vi "Fetch Measurement - Single point.vi"(8 "error in":errorcluster, 11 "Single point perform measurement":T1={"Source Ganged Session Out"={"Ganged Config"=enum."Series", "Session List"=[], "Session Mode"=[], "Channel"=[]}, "Load Ganged Session Out"={"Ganged Config"=enum."Series", "Session List"=[], "Session Mode"=[], "Channel"=[]}, "Source Measure Record Length"=0, "Load Measure Record Length"=0, "Measurement Results"={"dt"=[], "Source voltages"=[], "Source currents"=[], "Load voltages"=[], "Load currents"=[], "Ganged source voltages"=[], "Ganged source currents"=[], "Ganged load voltages"=[], "Ganged load currents"=[], "Mean values"=[], "Minimum values"=[], "Maximum values"=[], "Status"="", "Eload status"=""}, "Load Slave resource name"=[], "Load Master/Single resource name"="", "Source Slave resource name"=[], "Source Master/Single resource name"="", "Load ganged/single"=FALSE, "Source ganged/single"=FALSE, "Source channel name"="", "Load channel name"="", "Source session out"="", "Load session out"="", "Number of Eload used"=0, "Load Source ON/OFF"=enum."SOURCE ON", "Measurement timeout"=0.0}) -> (0 "error out":errorcluster, 3 "Single point perform measurement":T1={"Source Ganged Session Out"={"Ganged Config"=enum."Series", "Session List"=[], "Session Mode"=[], "Channel"=[]}, "Load Ganged Session Out"={"Ganged Config"=enum."Series", "Session List"=[], "Session Mode"=[], "Channel"=[]}, "Source Measure Record Length"=0, "Load Measure Record Length"=0, "Measurement Results"={"dt"=[], "Source voltages"=[], "Source currents"=[], "Load voltages"=[], "Load currents"=[], "Ganged source voltages"=[], "Ganged source currents"=[], "Ganged load voltages"=[], "Ganged load currents"=[], "Mean values"=[], "Minimum values"=[], "Maximum values"=[], "Status"="", "Eload status"=""}, "Load Slave resource name"=[], "Load Master/Single resource name"="", "Source Slave resource name"=[], "Source Master/Single resource name"="", "Load ganged/single"=FALSE, "Source ganged/single"=FALSE, "Source channel name"="", "Load channel name"="", "Source session out"="", "Load session out"="", "Number of Eload used"=0, "Load Source ON/OFF"=enum."SOURCE ON", "Measurement timeout"=0.0})   [LabVIEW 2021, in "Single Point_Channel Ganging.lvlib"]
doc: "This VI will fetch the measurement for different configuration for Single Point measurement"
uses:
  Single Point_Channel Ganging.lvlib
  Controls/Perform measurement-control.ctl
  shared subVIs/ctl/NIDCPower_channel_ganging - ctl - ganged session.ctl
  shared subVIs/ctl/NIDCPower_channel_ganging - ctl - ganged config.ctl
  shared subVIs/ctl/NIDCPower_channel_ganging - ctl - channel mode.ctl
  Measurement Results.ctl
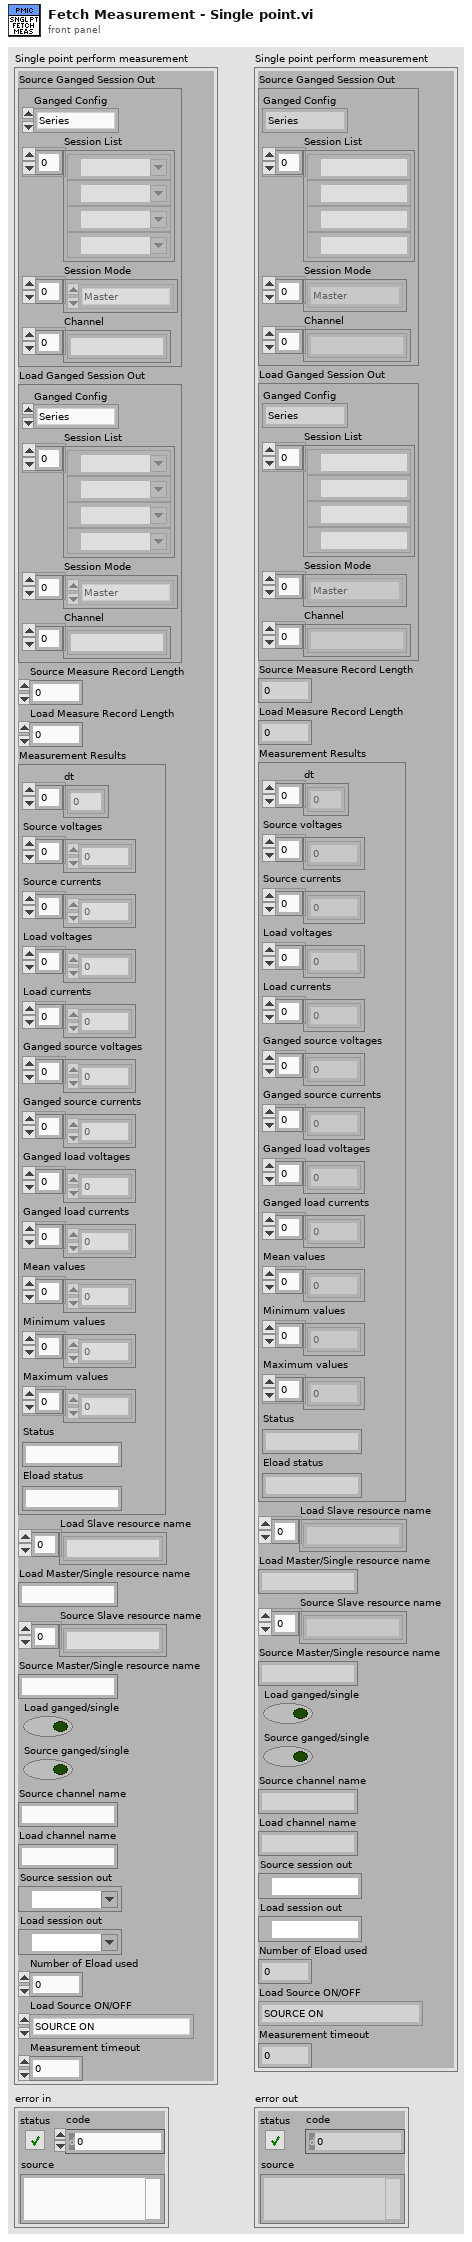
[diagram p1: front panel]
types:
  T1 = typedef "Single Point_Channel Ganging.lvlib/Perform measurement-control.ctl" = cluster{"Source Ganged Session Out":T2, "Load Ganged Session Out":T2, "Source Measure Record Length":i32, "Load Measure Record Length":i32, "Measurement Results":T5, "Load Slave resource name":string[], "Load Master/Single resource name":string, "Source Slave resource name":string[], "Source Master/Single resource name":string, "Load ganged/single":bool, "Source ganged/single":bool, "Source channel name":string, "Load channel name":string, "Source session out":refnum<k15>, "Load session out":refnum<k15>, "Number of Eload used":i32, "Load Source ON/OFF":enum16{"SOURCE AND LOAD OFF", "SOURCE ON", "LOAD ON", "SOURCE AND LOAD ON"}, "Measurement timeout":dbl}
  T2 = typedef "NIDCPower_channel_ganging - ctl - ganged session.ctl" = cluster{"Ganged Config":T3, "Session List":refnum<k15>[], "Session Mode":T4[], "Channel":string[]}
  T3 = typedef "NIDCPower_channel_ganging - ctl - ganged config.ctl" = enum32{"Series", "Parallel", "Manual"}
  T4 = typedef "NIDCPower_channel_ganging - ctl - channel mode.ctl" = enum32{"Master", "Slave", "Slave - Inverted"}
  T5 = typedef "Single Point_Channel Ganging.lvlib/Measurement Results.ctl" = cluster{"dt":dbl[], "Source voltages":dbl[], "Source currents":dbl[], "Load voltages":dbl[], "Load currents":dbl[], "Ganged source voltages":dbl[], "Ganged source currents":dbl[], "Ganged load voltages":dbl[], "Ganged load currents":dbl[], "Mean values":dbl[], "Minimum values":dbl[], "Maximum values":dbl[], "Status":string, "Eload status":string}
  T6 = enum16{"SOURCE AND LOAD OFF", "SOURCE ON", "LOAD ON", "SOURCE AND LOAD ON"}
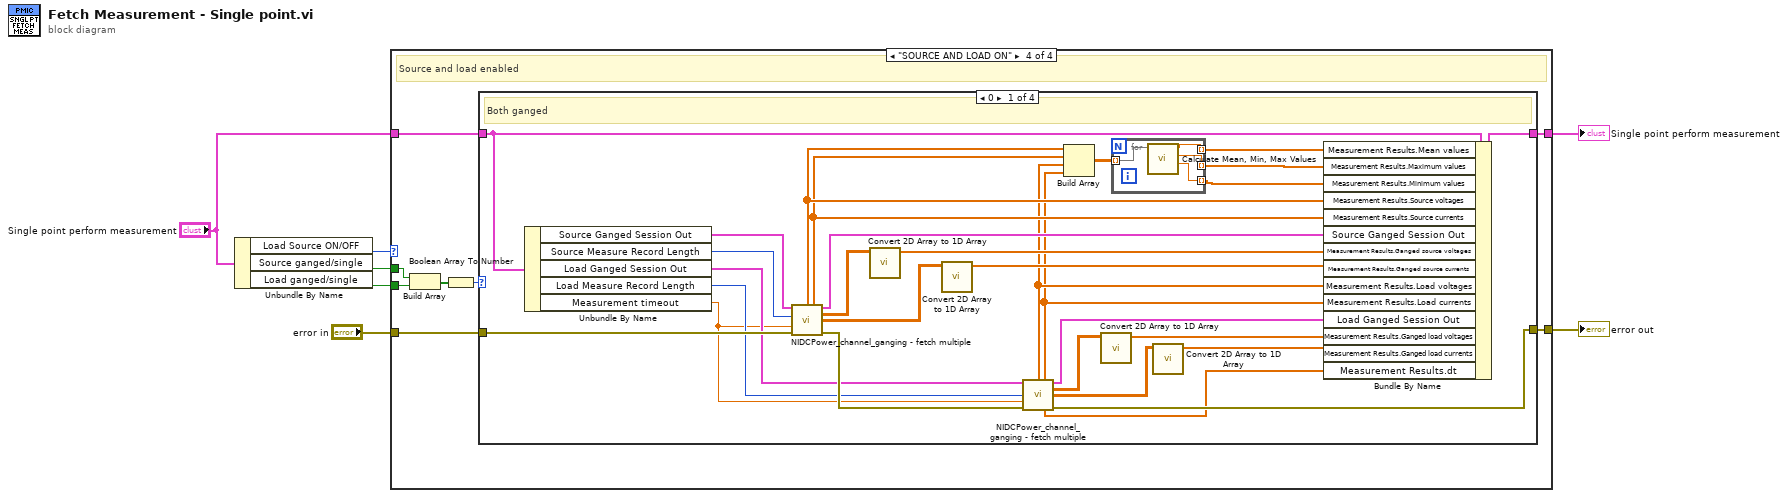
[diagram p0: block diagram]
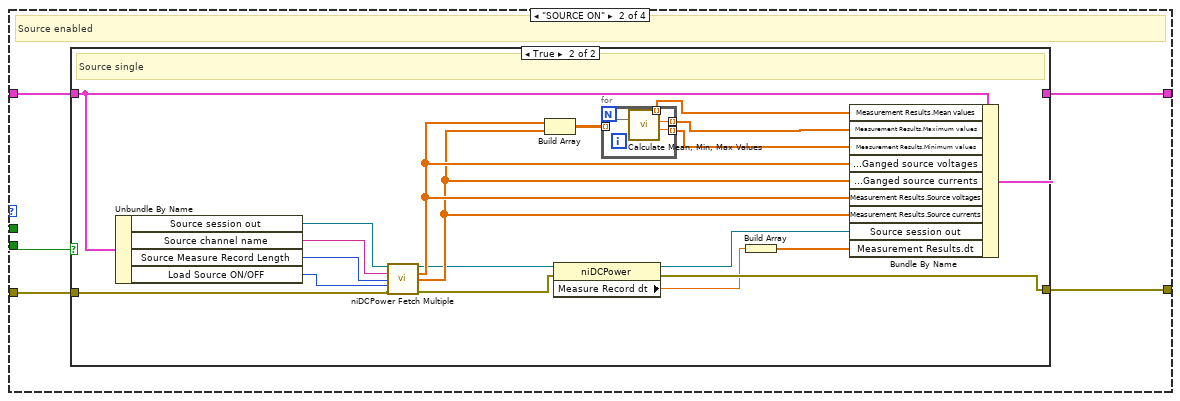
[diagram p3: hidden frame]
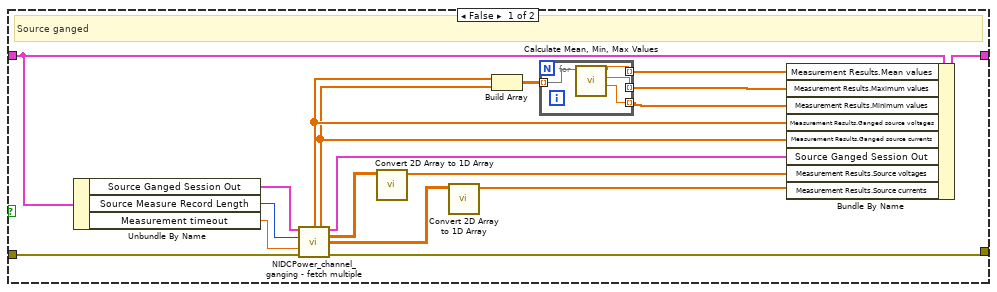
[diagram p4: hidden frame]
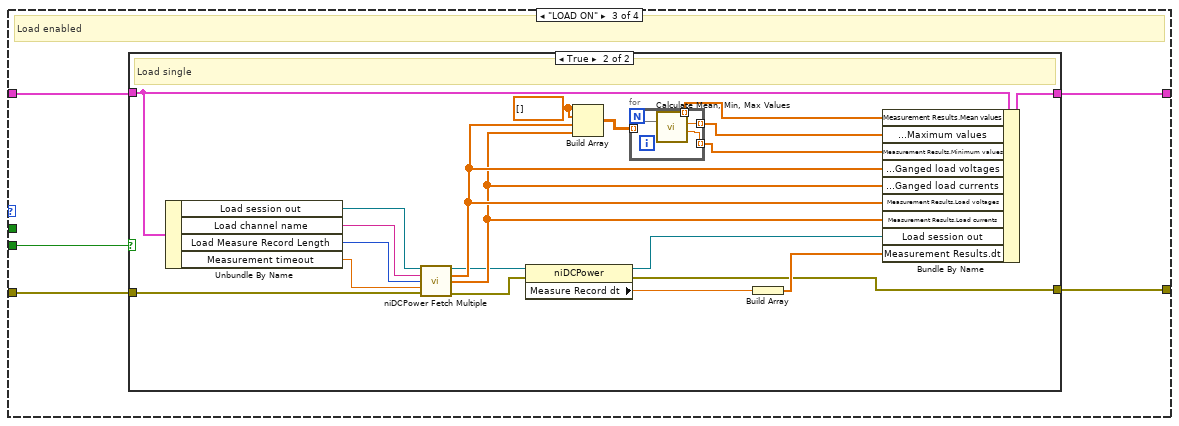
[diagram p5: hidden frame]
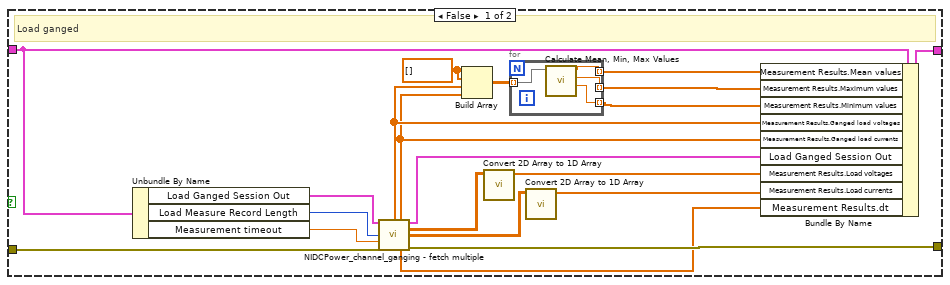
[diagram p6: hidden frame]
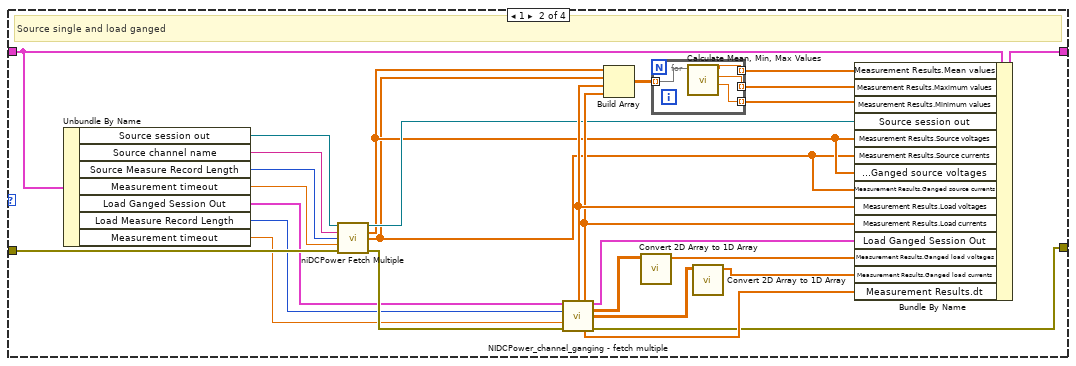
[diagram p7: hidden frame]
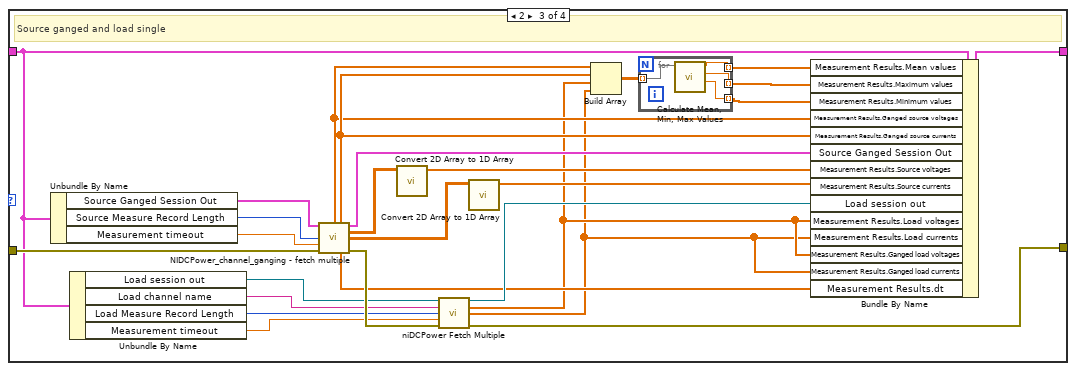
[diagram p8: hidden frame]
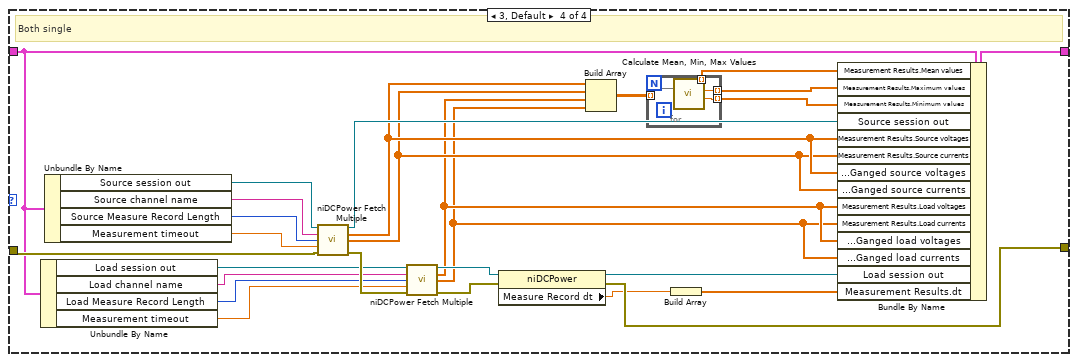
[diagram p9: hidden frame]
diagram:
  n1 = Unbundle By Name("Single point perform measurement") -> ("Load Source ON/OFF"=w5:T6, "Source ganged/single"=w6:bool, "Load ganged/single"=w7:bool)
  n2 = case shown="\"SOURCE AND LOAD ON\"" w5 {
    tunnel: "error in" -> [w8 w14 w64 w120]
    tunnel: [w9 w10 w60 w119] -> w2
    tunnel: [w8 w11 w61 w118] -> w3
    tunnel: "Single point perform measurement" -> [w9 w12 w63 w117]
    tunnel: w6 -> [_ w13 _ w115]
    tunnel: w7 -> [_ _ w62 w114]
    frame Default {
    }
    frame "SOURCE ON" {
      # "Source enabled"
      n3 = case shown="True" w13 {
        tunnel: w12 -> [w32 w55]
        tunnel: w14 -> [w30 w49]
        tunnel: [w29 w54] -> w10
        tunnel: [w16 w46] -> w11
        frame False {
          # "Source ganged"
          n4 = Unbundle By Name(w32) -> ("Source Ganged Session Out"=w31:T2, "Source Measure Record Length"=w27:i32, "Measurement timeout"=w15:dbl)
          n5 = call "NIDCPower_channel_ganging - fetch multiple.vi"("Ganged Session In"=w31, "Count"=w27, "timeout (1.0)"=w15, "error in (no error)"=w30) -> ("Ganged Voltage Measurement"=w22:dbl[], "Ganged Current Measurement"=w21:dbl[], "Ganged Session Out"=w28:T2, "voltage measurements"=w26:dbl[][], "current measurements"=w23:dbl[][], "error out"=w16:errorcluster)  [unwired: 4 in, 2 out]
          n6 = call "Convert 2D Array to 1D Array.vi"("Array in"=w26) -> ("Array out"=w25:dbl[])  [unwired: 10 in]
          n7 = call "Convert 2D Array to 1D Array.vi"("Array in"=w23) -> ("Array out"=w24:dbl[])  [unwired: 10 in]
          n8 = Build Array(w22, w21) -> (w20:dbl[][])
          n9 = for {
            tunnel: w20 -> [w36] mode=indexing
            tunnel: [w35] -> w19 mode=indexing
            tunnel: [w34] -> w18 mode=indexing
            tunnel: [w33] -> w17 mode=indexing
            n10 = call "Calculate Mean, Min, Max Values.vi"("Ganged Measurement"=w36) -> ("Min value"=w33:dbl, "Max value"=w34:dbl, "Mean value"=w35:dbl)  [unwired: 8 in]
          }
          n11 = Bundle By Name(cluster=w32, "Measurement Results.Mean values"=w19, "Measurement Results.Maximum values"=w18, "Measurement Results.Minimum values"=w17, "Measurement Results.Ganged source voltages"=w22, "Measurement Results.Ganged source currents"=w21, "Source Ganged Session Out"=w28, "Measurement Results.Source voltages"=w25, "Measurement Results.Source currents"=w24) -> (w29:T1)
        }
        frame True {
          # "Source single"
          n12 = Unbundle By Name(w55) -> ("Source session out"=w48:refnum<k15>, "Source channel name"=w39:string, "Source Measure Record Length"=w40:i32, "Load Source ON/OFF"=w37:T6)
          n13 = call <instrlib>:"niDCPower Fetch Multiple.vi"("instrument handle"=w48, "channel name"=w39, "count (1)"=w40, "timeout (1.0)"=w37, "error in (no error)"=w49) -> ("instrument handle out"=w42:refnum<k15>, "voltage measurements"=w47:dbl[], "current measurements"=w44:dbl[], "error out"=w43:errorcluster)  [unwired: 7 out]
          n14 = Build Array(w47, w44) -> (w53:dbl[][])
          n15 = property class="niDCPower"(reference=w42, error in=w43) -> (reference out=w38:refnum<k15>, error out=w46:errorcluster, "Measure Record dt"=w45:dbl)
          n16 = for {
            tunnel: w53 -> [w59] mode=indexing
            tunnel: [w58] -> w52 mode=indexing
            tunnel: [w57] -> w51 mode=indexing
            tunnel: [w56] -> w50 mode=indexing
            n17 = call "Calculate Mean, Min, Max Values.vi"("Ganged Measurement"=w59) -> ("Min value"=w56:dbl, "Max value"=w57:dbl, "Mean value"=w58:dbl)  [unwired: 8 in]
          }
          n18 = Build Array(w45) -> (w41:dbl[])
          n19 = Bundle By Name(cluster=w55, "Measurement Results.Mean values"=w52, "Measurement Results.Maximum values"=w51, "Measurement Results.Minimum values"=w50, "Measurement Results.Ganged source voltages"=w47, "Measurement Results.Ganged source currents"=w44, "Measurement Results.Source voltages"=w47, "Measurement Results.Source currents"=w44, "Source session out"=w38, "Measurement Results.dt"=w41) -> (w54:T1)
        }
      }
    }
    frame "LOAD ON" {
      # "Load enabled"
      n20 = case shown="True" w62 {
        tunnel: w63 -> [w84 w104]
        tunnel: w64 -> [w68 w93]
        tunnel: [w82 w103] -> w60
        tunnel: [w81 w90] -> w61
        frame False {
          w65 = dbl[] [] ("element")
          # "Load ganged"
          n21 = Unbundle By Name(w84) -> ("Load Ganged Session Out"=w83:T2, "Load Measure Record Length"=w66:i32, "Measurement timeout"=w67:dbl)
          n22 = call "NIDCPower_channel_ganging - fetch multiple.vi"("Ganged Session In"=w83, "Count"=w66, "timeout (1.0)"=w67, "error in (no error)"=w68) -> ("Ganged Voltage Measurement"=w74:dbl[], "Ganged Current Measurement"=w73:dbl[], "Ganged Session Out"=w80:T2, "voltage measurements"=w78:dbl[][], "current measurements"=w76:dbl[][], "Measure Record dt"=w79:dbl[], "error out"=w81:errorcluster)  [unwired: 4 in, 1 out]
          n23 = Build Array(w65, w65, w74, w73) -> (w72:dbl[][])
          n24 = call "Convert 2D Array to 1D Array.vi"("Array in"=w78) -> ("Array out"=w77:dbl[])  [unwired: 10 in]
          n25 = for {
            tunnel: w72 -> [w88] mode=indexing
            tunnel: [w87] -> w71 mode=indexing
            tunnel: [w86] -> w70 mode=indexing
            tunnel: [w85] -> w69 mode=indexing
            n26 = call "Calculate Mean, Min, Max Values.vi"("Ganged Measurement"=w88) -> ("Min value"=w85:dbl, "Max value"=w86:dbl, "Mean value"=w87:dbl)  [unwired: 8 in]
          }
          n27 = call "Convert 2D Array to 1D Array.vi"("Array in"=w76) -> ("Array out"=w75:dbl[])  [unwired: 10 in]
          n28 = Bundle By Name(cluster=w84, "Measurement Results.Mean values"=w71, "Measurement Results.Maximum values"=w70, "Measurement Results.Minimum values"=w69, "Measurement Results.Ganged load voltages"=w74, "Measurement Results.Ganged load currents"=w73, "Load Ganged Session Out"=w80, "Measurement Results.Load voltages"=w77, "Measurement Results.Load currents"=w75, "Measurement Results.dt"=w79) -> (w82:T1)
        }
        frame True {
          w89 = dbl[] [] ("element")
          # "Load single"
          n29 = Unbundle By Name(w104) -> ("Load session out"=w108:refnum<k15>, "Load channel name"=w107:string, "Load Measure Record Length"=w94:i32, "Measurement timeout"=w91:dbl)
          n30 = call <instrlib>:"niDCPower Fetch Multiple.vi"("instrument handle"=w108, "channel name"=w107, "count (1)"=w94, "timeout (1.0)"=w91, "error in (no error)"=w93) -> ("instrument handle out"=w97:refnum<k15>, "voltage measurements"=w106:dbl[], "current measurements"=w105:dbl[], "error out"=w98:errorcluster)  [unwired: 7 out]
          n31 = property class="niDCPower"(reference=w97, error in=w98) -> (reference out=w92:refnum<k15>, error out=w90:errorcluster, "Measure Record dt"=w96:dbl)
          n32 = Build Array(w89, w89, w106, w105) -> (w102:dbl[][])
          n33 = for {
            tunnel: w102 -> [w112] mode=indexing
            tunnel: [w111] -> w101 mode=indexing
            tunnel: [w110] -> w100 mode=indexing
            tunnel: [w109] -> w99 mode=indexing
            n34 = call "Calculate Mean, Min, Max Values.vi"("Ganged Measurement"=w112) -> ("Min value"=w109:dbl, "Max value"=w110:dbl, "Mean value"=w111:dbl)  [unwired: 8 in]
          }
          n35 = Build Array(w96) -> (w95:dbl[])
          n36 = Bundle By Name(cluster=w104, "Measurement Results.Mean values"=w101, "Measurement Results.Maximum values"=w100, "Measurement Results.Minimum values"=w99, "Measurement Results.Ganged load voltages"=w106, "Measurement Results.Ganged load currents"=w105, "Measurement Results.Load voltages"=w106, "Measurement Results.Load currents"=w105, "Load session out"=w92, "Measurement Results.dt"=w95) -> (w103:T1)
        }
      }
    }
    frame "SOURCE AND LOAD ON" {
      # "Source and load enabled"
      n37 = Build Array(w115, w114) -> (w116:bool[])
      n38 = Boolean Array To Number(Boolean array=w116) -> (number=w113:u32)
      n39 = case shown="0" w113 {
        tunnel: w117 -> [w149 w160 w192 w228]
        tunnel: w120 -> [w146 w167 w199 w236]
        tunnel: [w144 w168 w198 w242] -> w119
        tunnel: [w143 w156 w196 w231] -> w118
        frame 0 {
          # "Both ganged"
          n40 = Unbundle By Name(w149) -> ("Source Ganged Session Out"=w148:T2, "Source Measure Record Length"=w123:i32, "Load Ganged Session Out"=w145:T2, "Load Measure Record Length"=w122:i32, "Measurement timeout"=w121:dbl)
          n41 = call "NIDCPower_channel_ganging - fetch multiple.vi"("Ganged Session In"=w148, "Count"=w123, "timeout (1.0)"=w121, "error in (no error)"=w146) -> ("Ganged Voltage Measurement"=w131:dbl[], "Ganged Current Measurement"=w130:dbl[], "Ganged Session Out"=w142:T2, "voltage measurements"=w139:dbl[][], "current measurements"=w136:dbl[][], "error out"=w147:errorcluster)  [unwired: 4 in, 2 out]
          n42 = call "Convert 2D Array to 1D Array.vi"("Array in"=w139) -> ("Array out"=w138:dbl[])  [unwired: 10 in]
          n43 = call "Convert 2D Array to 1D Array.vi"("Array in"=w136) -> ("Array out"=w137:dbl[])  [unwired: 10 in]
          n44 = call "NIDCPower_channel_ganging - fetch multiple.vi"("Ganged Session In"=w145, "Count"=w122, "timeout (1.0)"=w121, "error in (no error)"=w147) -> ("Ganged Voltage Measurement"=w129:dbl[], "Ganged Current Measurement"=w128:dbl[], "Ganged Session Out"=w141:T2, "voltage measurements"=w135:dbl[][], "current measurements"=w133:dbl[][], "Measure Record dt"=w140:dbl[], "error out"=w143:errorcluster)  [unwired: 4 in, 1 out]
          n45 = Build Array(w131, w130, w129, w128) -> (w127:dbl[][])
          n46 = call "Convert 2D Array to 1D Array.vi"("Array in"=w135) -> ("Array out"=w134:dbl[])  [unwired: 10 in]
          n47 = for {
            tunnel: w127 -> [w153] mode=indexing
            tunnel: [w152] -> w126 mode=indexing
            tunnel: [w151] -> w125 mode=indexing
            tunnel: [w150] -> w124 mode=indexing
            n48 = call "Calculate Mean, Min, Max Values.vi"("Ganged Measurement"=w153) -> ("Min value"=w150:dbl, "Max value"=w151:dbl, "Mean value"=w152:dbl)  [unwired: 8 in]
          }
          n49 = call "Convert 2D Array to 1D Array.vi"("Array in"=w133) -> ("Array out"=w132:dbl[])  [unwired: 10 in]
          n50 = Bundle By Name(cluster=w149, "Measurement Results.Mean values"=w126, "Measurement Results.Maximum values"=w125, "Measurement Results.Minimum values"=w124, "Measurement Results.Source voltages"=w131, "Measurement Results.Source currents"=w130, "Source Ganged Session Out"=w142, "Measurement Results.Ganged source voltages"=w138, "Measurement Results.Ganged source currents"=w137, "Measurement Results.Load voltages"=w129, "Measurement Results.Load currents"=w128, "Load Ganged Session Out"=w141, "Measurement Results.Ganged load voltages"=w134, "Measurement Results.Ganged load currents"=w132, "Measurement Results.dt"=w140) -> (w144:T1)
        }
        frame 1 {
          # "Source single and load ganged"
          n51 = Unbundle By Name(w160) -> ("Source session out"=w165:refnum<k15>, "Source channel name"=w162:string, "Source Measure Record Length"=w164:i32, "Measurement timeout"=w159:dbl, "Load Ganged Session Out"=w158:T2, "Load Measure Record Length"=w161:i32, "Measurement timeout"=w157:dbl)
          n52 = call <instrlib>:"niDCPower Fetch Multiple.vi"("instrument handle"=w165, "channel name"=w162, "count (1)"=w164, "timeout (1.0)"=w159, "error in (no error)"=w167) -> ("instrument handle out"=w163:refnum<k15>, "voltage measurements"=w155:dbl[], "current measurements"=w154:dbl[], "error out"=w166:errorcluster)  [unwired: 7 out]
          n53 = call "NIDCPower_channel_ganging - fetch multiple.vi"("Ganged Session In"=w158, "Count"=w161, "timeout (1.0)"=w157, "error in (no error)"=w166) -> ("Ganged Voltage Measurement"=w174:dbl[], "Ganged Current Measurement"=w173:dbl[], "Ganged Session Out"=w180:T2, "voltage measurements"=w178:dbl[][], "current measurements"=w176:dbl[][], "Measure Record dt"=w179:dbl[], "error out"=w156:errorcluster)  [unwired: 4 in, 1 out]
          n54 = Build Array(w155, w154, w174, w173) -> (w172:dbl[][])
          n55 = call "Convert 2D Array to 1D Array.vi"("Array in"=w178) -> ("Array out"=w177:dbl[])  [unwired: 10 in]
          n56 = for {
            tunnel: w172 -> [w184] mode=indexing
            tunnel: [w183] -> w171 mode=indexing
            tunnel: [w182] -> w170 mode=indexing
            tunnel: [w181] -> w169 mode=indexing
            n57 = call "Calculate Mean, Min, Max Values.vi"("Ganged Measurement"=w184) -> ("Min value"=w181:dbl, "Max value"=w182:dbl, "Mean value"=w183:dbl)  [unwired: 8 in]
          }
          n58 = call "Convert 2D Array to 1D Array.vi"("Array in"=w176) -> ("Array out"=w175:dbl[])  [unwired: 10 in]
          n59 = Bundle By Name(cluster=w160, "Measurement Results.Mean values"=w171, "Measurement Results.Maximum values"=w170, "Measurement Results.Minimum values"=w169, "Source session out"=w163, "Measurement Results.Source voltages"=w155, "Measurement Results.Source currents"=w154, "Measurement Results.Ganged source voltages"=w155, "Measurement Results.Ganged source currents"=w154, "Measurement Results.Load voltages"=w174, "Measurement Results.Load currents"=w173, "Load Ganged Session Out"=w180, "Measurement Results.Ganged load voltages"=w177, "Measurement Results.Ganged load currents"=w175, "Measurement Results.dt"=w179) -> (w168:T1)
        }
        frame 2 {
          # "Source ganged and load single"
          n60 = Unbundle By Name(w192) -> ("Source Ganged Session Out"=w200:T2, "Source Measure Record Length"=w194:i32, "Measurement timeout"=w187:dbl)
          n61 = Unbundle By Name(w192) -> ("Load session out"=w191:refnum<k15>, "Load channel name"=w190:string, "Load Measure Record Length"=w189:i32, "Measurement timeout"=w188:dbl)
          n62 = call "NIDCPower_channel_ganging - fetch multiple.vi"("Ganged Session In"=w200, "Count"=w194, "timeout (1.0)"=w187, "error in (no error)"=w199) -> ("Ganged Voltage Measurement"=w206:dbl[], "Ganged Current Measurement"=w207:dbl[], "Ganged Session Out"=w201:T2, "voltage measurements"=w202:dbl[][], "current measurements"=w205:dbl[][], "Measure Record dt"=w193:dbl[], "error out"=w197:errorcluster)  [unwired: 4 in, 1 out]
          n63 = call "Convert 2D Array to 1D Array.vi"("Array in"=w202) -> ("Array out"=w203:dbl[])  [unwired: 10 in]
          n64 = call <instrlib>:"niDCPower Fetch Multiple.vi"("instrument handle"=w191, "channel name"=w190, "count (1)"=w189, "timeout (1.0)"=w188, "error in (no error)"=w197) -> ("instrument handle out"=w195:refnum<k15>, "voltage measurements"=w186:dbl[], "current measurements"=w185:dbl[], "error out"=w196:errorcluster)  [unwired: 7 out]
          n65 = call "Convert 2D Array to 1D Array.vi"("Array in"=w205) -> ("Array out"=w204:dbl[])  [unwired: 10 in]
          n66 = Build Array(w206, w207, w186, w185) -> (w208:dbl[][])
          n67 = for {
            tunnel: w208 -> [w215] mode=indexing
            tunnel: [w214] -> w209 mode=indexing
            tunnel: [w213] -> w210 mode=indexing
            tunnel: [w212] -> w211 mode=indexing
            n68 = call "Calculate Mean, Min, Max Values.vi"("Ganged Measurement"=w215) -> ("Min value"=w212:dbl, "Max value"=w213:dbl, "Mean value"=w214:dbl)  [unwired: 8 in]
          }
          n69 = Bundle By Name(cluster=w192, "Measurement Results.Mean values"=w209, "Measurement Results.Maximum values"=w210, "Measurement Results.Minimum values"=w211, "Measurement Results.Ganged source voltages"=w206, "Measurement Results.Ganged source currents"=w207, "Source Ganged Session Out"=w201, "Measurement Results.Source voltages"=w203, "Measurement Results.Source currents"=w204, "Load session out"=w195, "Measurement Results.Load voltages"=w186, "Measurement Results.Load currents"=w185, "Measurement Results.Ganged load voltages"=w186, "Measurement Results.Ganged load currents"=w185, "Measurement Results.dt"=w193) -> (w198:T1)
        }
        frame 3, Default {
          # "Both single"
          n70 = Unbundle By Name(w228) -> ("Load session out"=w227:refnum<k15>, "Load channel name"=w226:string, "Load Measure Record Length"=w225:i32, "Measurement timeout"=w220:dbl)
          n71 = Unbundle By Name(w228) -> ("Source session out"=w235:refnum<k15>, "Source channel name"=w223:string, "Source Measure Record Length"=w224:i32, "Measurement timeout"=w221:dbl)
          n72 = call <instrlib>:"niDCPower Fetch Multiple.vi"("instrument handle"=w235, "channel name"=w223, "count (1)"=w224, "timeout (1.0)"=w221, "error in (no error)"=w236) -> ("instrument handle out"=w234:refnum<k15>, "voltage measurements"=w219:dbl[], "current measurements"=w218:dbl[], "error out"=w237:errorcluster)  [unwired: 7 out]
          n73 = call <instrlib>:"niDCPower Fetch Multiple.vi"("instrument handle"=w227, "channel name"=w226, "count (1)"=w225, "timeout (1.0)"=w220, "error in (no error)"=w237) -> ("instrument handle out"=w232:refnum<k15>, "voltage measurements"=w217:dbl[], "current measurements"=w216:dbl[], "error out"=w233:errorcluster)  [unwired: 7 out]
          n74 = property class="niDCPower"(reference=w232, error in=w233) -> (reference out=w222:refnum<k15>, error out=w231:errorcluster, "Measure Record dt"=w230:dbl)
          n75 = Build Array(w219, w218, w217, w216) -> (w241:dbl[][])
          n76 = for {
            tunnel: w241 -> [w246] mode=indexing
            tunnel: [w245] -> w240 mode=indexing
            tunnel: [w244] -> w239 mode=indexing
            tunnel: [w243] -> w238 mode=indexing
            n77 = call "Calculate Mean, Min, Max Values.vi"("Ganged Measurement"=w246) -> ("Min value"=w243:dbl, "Max value"=w244:dbl, "Mean value"=w245:dbl)  [unwired: 8 in]
          }
          n78 = Build Array(w230) -> (w229:dbl[])
          n79 = Bundle By Name(cluster=w228, "Measurement Results.Mean values"=w240, "Measurement Results.Maximum values"=w239, "Measurement Results.Minimum values"=w238, "Source session out"=w234, "Measurement Results.Source voltages"=w219, "Measurement Results.Source currents"=w218, "Measurement Results.Ganged source voltages"=w219, "Measurement Results.Ganged source currents"=w218, "Measurement Results.Load voltages"=w217, "Measurement Results.Load currents"=w216, "Measurement Results.Ganged load voltages"=w217, "Measurement Results.Ganged load currents"=w216, "Load session out"=w222, "Measurement Results.dt"=w229) -> (w242:T1)
        }
      }
    }
  }
  "error out" <- w3
  "Single point perform measurement" <- w2
